vi "Begin.vi"(8 "error in":errorcluster) -> (0 "error out":errorcluster)   [LabVIEW 2020]
doc: "Called before other user functions, this VI is expected to open initial I/O refnums, load in file data, and do all program initialization. Notice that the <B>error out</B> terminal is simply used for data flow. Wiring it to other structures or subVIs ensures that this VI runs first."
uses:
  <vilib>/Rock Robotics/WPI/DriverStation/WPI_DriverStationRobotMode2.ctl
  <vilib>/Rock Robotics/WPI/Joystick/WPI_JoystickDeviceEnum.ctl
  <vilib>/Rock Robotics/WPI/ThirdParty/REV Robotics/REVLib/Typedef/Spark MAX Sensor Type.ctl
  Robot Global Data.vi
  <vilib>/Rock Robotics/Network Tables/NT Write String Array.vi
panel:
  in  "Steering BR PIDF":T1={"P Gain"=0.0, "I Gain"=0.0, "D Gain"=0.0, "F Gain"=0.0, "I Zone"=0.0, "Min Output"=-1.0, "Max Output"=1.0}
  in  "Steering BL PIDF":T1={"P Gain"=0.0, "I Gain"=0.0, "D Gain"=0.0, "F Gain"=0.0, "I Zone"=0.0, "Min Output"=-1.0, "Max Output"=1.0}
  in  "Steering FR PIDF":T1={"P Gain"=0.0, "I Gain"=0.0, "D Gain"=0.0, "F Gain"=0.0, "I Zone"=0.0, "Min Output"=-1.0, "Max Output"=1.0}
  in  "Steering FL PIDF":T1={"P Gain"=0.0, "I Gain"=0.0, "D Gain"=0.0, "F Gain"=0.0, "I Zone"=0.0, "Min Output"=-1.0, "Max Output"=1.0}
  in  "FR Zero":dbl
  in  "FL Zero":dbl
  in  "Reset Encoders":bool
  in  "BL Zero":dbl
  in  "BR Zero":dbl
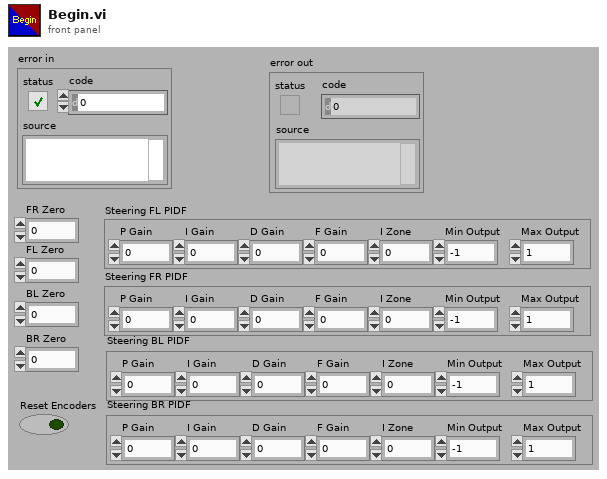
[diagram p1: front panel]
types:
  T1 = cluster{"P Gain":dbl, "I Gain":dbl, "D Gain":dbl, "F Gain":dbl, "I Zone":dbl, "Min Output":dbl, "Max Output":dbl}
  T2 = typedef "Spark MAX Sensor Type.ctl" = enum16{"No Sensor", "Hall Sensor", "Encoder", "-Not Available-", "Analog", "Alternate Encoder", "Duty Cycle"}
  T3 = typedef "WPI_JoystickDeviceEnum.ctl" = enum16{"USB 0", "USB 1", "USB 2", "USB 3", "USB 4", "USB 5"}
  T4 = typedef "WPI_DriverStationRobotMode2.ctl" = enum16{"Autonomous Disabled", "Autonomous Enabled", "Teleop Disabled", "Teleop Enabled", "Disconnected", "Finish", "Test Disabled", "Test Enabled", "Emergency Stopped"}
  T5 = typedef "WPI_JoystickDevRef.ctl" = cluster{"Device":T3}
  T6 = typedef "WPI_MotorControlDeviceRef.ctl" = cluster{"DeviceStatus":errorcluster, "Type":T7, "PWM":cluster{"PWM Channel":T8, "DeadBand":T9}, "CAN":cluster{"Device Number":u8, "SetOutput VI Ref":variant, "GetOutput VI Ref":variant, "Enable VI Ref":variant, "Disable VI Ref":variant, "Data":variant}, "Invert":bool, "DIO PWM":cluster{"PWM \"Enable\" Channel":T8, "DIOChannel":T10, "PWM Rate":dbl}}
  T7 = typedef "WPI_MotorControlType.ctl" = enum16{"PWM", "CAN", "DIO PWM"}
  T8 = typedef "FPGA_DIOPWMChannel.ctl" = enum8{"PWM 0", "PWM 1", "PWM 2", "PWM 3", "PWM 4", "PWM 5", "PWM 6", "PWM 7", "PWM 8", "PWM 9", "PWM MXP 0", "PWM MXP 1", "PWM MXP 2", "PWM MXP 3", "PWM MXP 4", "PWM MXP 5", "PWM MXP 6", "PWM MXP 7", "PWM MXP 8", "PWM MXP 9", "Invalid"}
  T9 = typedef "WPI_PWMDeadband.ctl" = cluster{"Name":string, "maxPositivePwm":i32, "minPositivePwm":i32, "centerPwm":i32, "maxNegativePwm":i32, "minNegativePwm":i32, "angularRange":u16}
  T10 = typedef "FPGA_DIOChannel.ctl" = enum8{"DIO 0", "DIO 1", "DIO 2", "DIO 3", "DIO 4", "DIO 5", "DIO 6", "DIO 7", "DIO 8", "DIO 9", "DIO MXP 0", "DIO MXP 1", "DIO MXP 2", "DIO MXP 3", "DIO MXP 4", "DIO MXP 5", "DIO MXP 6", "DIO MXP 7", "DIO MXP 8", "DIO MXP 9", "DIO MXP 10", "DIO MXP 11", "DIO MXP 12", "DIO MXP 13", "DIO MXP 14", "DIO MXP 15", "SPI Port CS1", "SPI Port CS2", "SPI Port CS3", "SPI Port MISO", "SPI Port MOSI", "Invalid"}
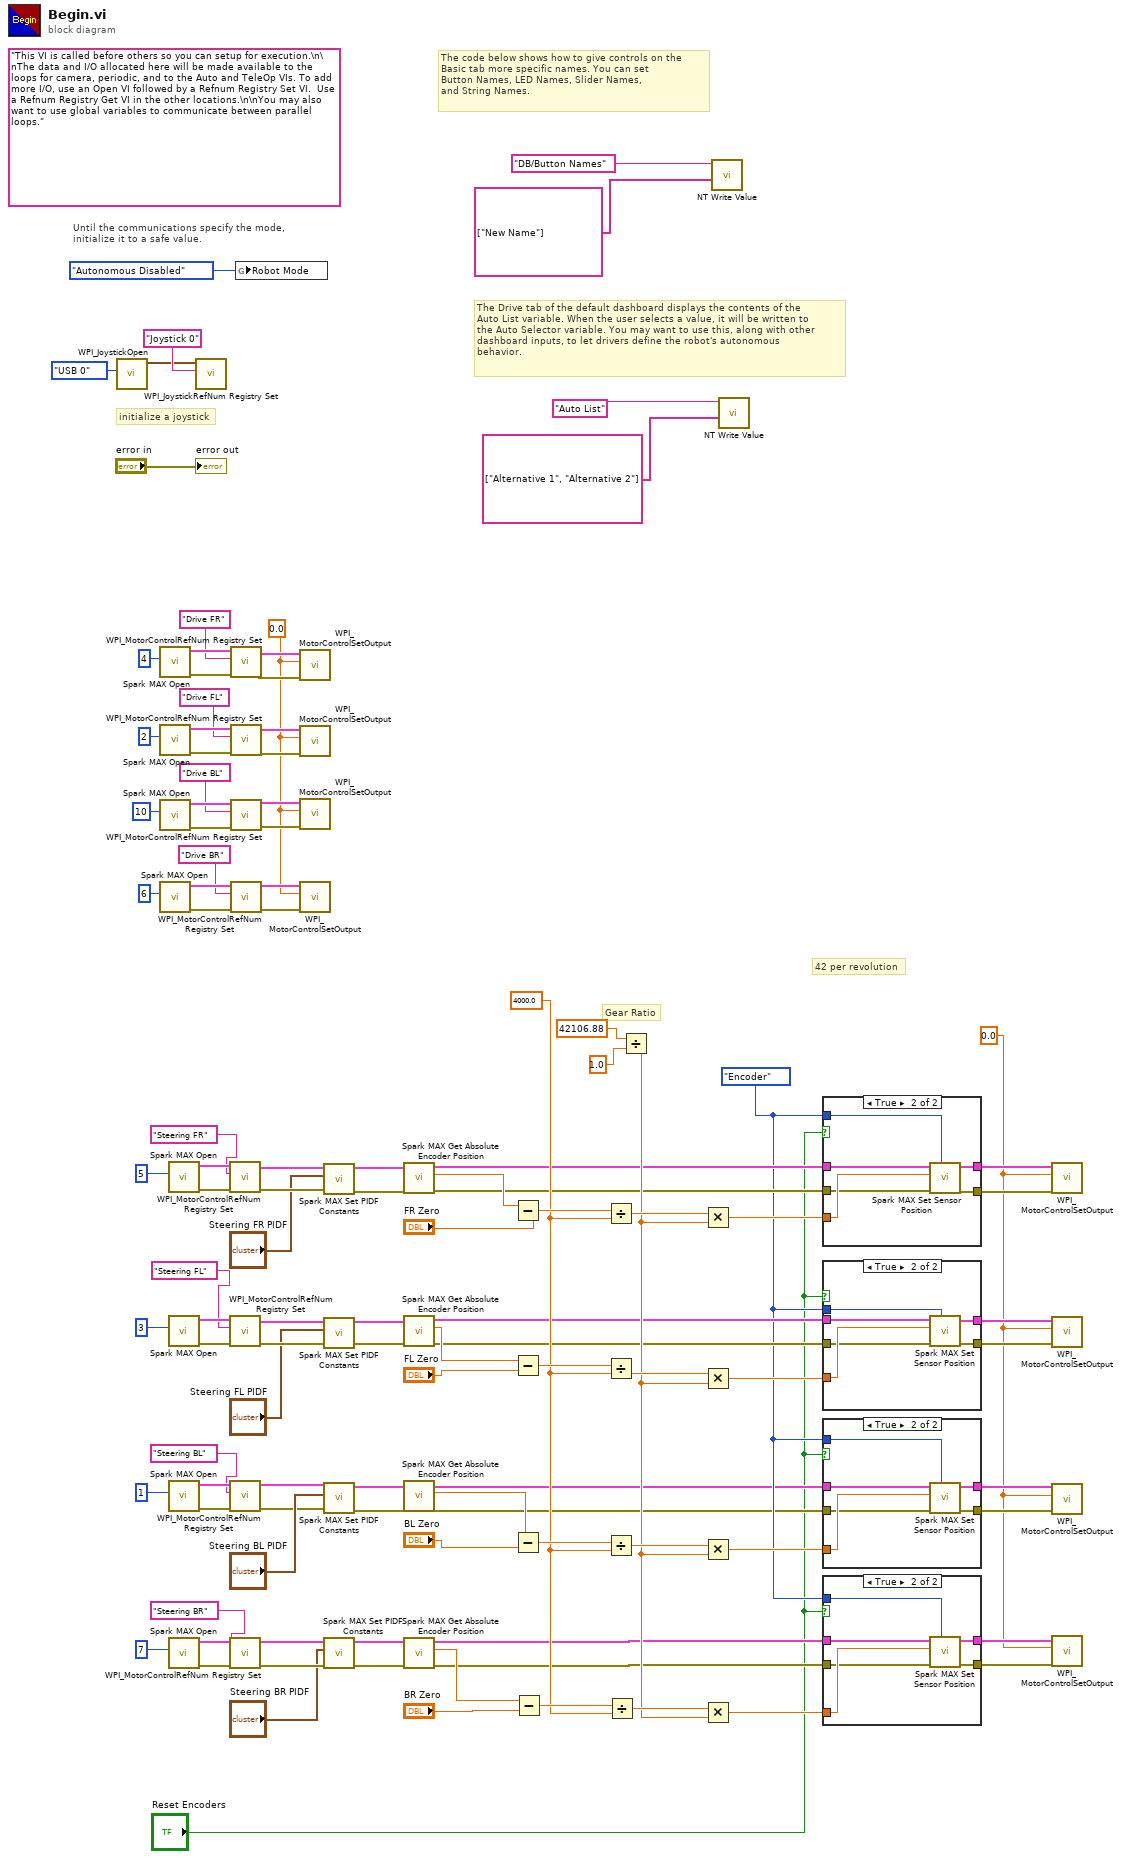
[diagram p0: block diagram]
diagram:
  w20 = 0.0 ("Output")
  w32 = Spark_MAX_Sensor_Type."Encoder" ("Sensor Type (Hall Sensor)")
  w43 = 4000.0 ("y")
  w79 = 0.0 ("Output")
  (unwired) "This VI is called before others so you can setup for execution.\n\nThe data and I/O allocated here will be made available to the loops for camera, periodic, and to the Auto and TeleOp VIs. To add more I/O, use an Open VI followed by a Refnum Registry Set VI.  Use a Refnum Registry Get VI in the other locations.\n\nYou may also want to use global variables to communicate between parallel loops."
  # "42 per revolution"
  # "Gear Ratio"
  # "The Drive tab of the default dashboard displays the contents of the\nAuto List variable. When the user selects a value, it will be written to\nthe Auto Selector variable. You may want to use this, along with other\ndashboard inputs, to let drivers define the robot's autonomous\nbehavior."
  # "The code below shows how to give controls on the\nBasic tab more specific names. You can set\nButton Names, LED Names, Slider Names,\nand String Names."
  # "initialize a joystick"
  # "Until the communications specify the mode,\ninitialize it to a safe value."
  n1 = call <vilib>:"WPI_JoystickOpen.vi"("JoystickDevice"=WPI_JoystickDeviceEnum."USB 0") -> ("JoystickDevRef"=w110:T5)  [unwired: 10 in]
  n2 = call <vilib>:"Spark MAX Open.vi"("Device Number"=u8 4) -> ("error out"=w102:errorcluster, "MotorControlDeviceRef"=w103:T6)  [unwired: 9 in]
  n3 = call <vilib>:"Spark MAX Open.vi"("Device Number"=u8 2) -> ("error out"=w98:errorcluster, "MotorControlDeviceRef"=w99:T6)  [unwired: 9 in]
  n4 = call <vilib>:"Spark MAX Open.vi"("Device Number"=u8 10) -> ("error out"=w94:errorcluster, "MotorControlDeviceRef"=w95:T6)  [unwired: 9 in]
  n5 = call <vilib>:"Spark MAX Open.vi"("Device Number"=u8 6) -> ("error out"=w90:errorcluster, "MotorControlDeviceRef"=w91:T6)  [unwired: 9 in]
  n6 = call <vilib>:"Spark MAX Open.vi"("Device Number"=u8 5) -> ("error out"=w77:errorcluster, "MotorControlDeviceRef"=w78:T6)  [unwired: 9 in]
  n7 = call <vilib>:"Spark MAX Open.vi"("Device Number"=u8 3) -> ("error out"=w73:errorcluster, "MotorControlDeviceRef"=w74:T6)  [unwired: 9 in]
  n8 = call <vilib>:"Spark MAX Open.vi"("Device Number"=u8 1) -> ("error out"=w69:errorcluster, "MotorControlDeviceRef"=w70:T6)  [unwired: 9 in]
  n9 = call <vilib>:"Spark MAX Open.vi"("Device Number"=u8 7) -> ("error out"=w65:errorcluster, "MotorControlDeviceRef"=w66:T6)  [unwired: 9 in]
  n10 = call <vilib>:"WPI_JoystickRefNum Registry Set.vi"("refnum name"="Joystick 0", "JoystickDevRef"=w110) -> ()  [unwired: 8 in, 2 out]
  n11 = call <vilib>:"WPI_MotorControlRefNum Registry Set.vi"("error in (no error)"=w77, "refnum name"="Steering FR", "MotorControlDevRef"=w78) -> ("error out"=w14:errorcluster, "MotorControlDevRef"=w15:T6)  [unwired: 7 in]
  n12 = call <vilib>:"WPI_MotorControlRefNum Registry Set.vi"("error in (no error)"=w73, "refnum name"="Steering FL", "MotorControlDevRef"=w74) -> ("error out"=w27:errorcluster, "MotorControlDevRef"=w17:T6)  [unwired: 7 in]
  n13 = call <vilib>:"WPI_MotorControlRefNum Registry Set.vi"("error in (no error)"=w69, "refnum name"="Steering BL", "MotorControlDevRef"=w70) -> ("error out"=w8:errorcluster, "MotorControlDevRef"=w9:T6)  [unwired: 7 in]
  n14 = call <vilib>:"WPI_MotorControlRefNum Registry Set.vi"("error in (no error)"=w65, "refnum name"="Steering BR", "MotorControlDevRef"=w66) -> ("error out"=w3:errorcluster, "MotorControlDevRef"=w2:T6)  [unwired: 7 in]
  n15 = call <vilib>:"WPI_MotorControlRefNum Registry Set.vi"("error in (no error)"=w102, "refnum name"="Drive FR", "MotorControlDevRef"=w103) -> ("error out"=w85:errorcluster, "MotorControlDevRef"=w84:T6)  [unwired: 7 in]
  n16 = call <vilib>:"WPI_MotorControlRefNum Registry Set.vi"("error in (no error)"=w98, "refnum name"="Drive FL", "MotorControlDevRef"=w99) -> ("error out"=w86:errorcluster, "MotorControlDevRef"=w87:T6)  [unwired: 7 in]
  n17 = call <vilib>:"WPI_MotorControlRefNum Registry Set.vi"("error in (no error)"=w94, "refnum name"="Drive BL", "MotorControlDevRef"=w95) -> ("error out"=w82:errorcluster, "MotorControlDevRef"=w83:T6)  [unwired: 7 in]
  n18 = call <vilib>:"WPI_MotorControlRefNum Registry Set.vi"("error in (no error)"=w90, "refnum name"="Drive BR", "MotorControlDevRef"=w91) -> ("error out"=w81:errorcluster, "MotorControlDevRef"=w80:T6)  [unwired: 7 in]
  n19 = global write "Robot Global Data.vi" "Robot Mode"(WPI_DriverStationRobotMode2."Autonomous Disabled" ("Robot Mode")) -> ()
  n20 = call <vilib>:"WPI_MotorControlSetOutput.vi"("error in (no error)"=w85, "Output"=w79, "MotorControlDevRef"=w84) -> ()  [unwired: 6 in, 3 out]
  n21 = call <vilib>:"WPI_MotorControlSetOutput.vi"("error in (no error)"=w86, "Output"=w79, "MotorControlDevRef"=w87) -> ()  [unwired: 6 in, 3 out]
  n22 = call <vilib>:"WPI_MotorControlSetOutput.vi"("error in (no error)"=w82, "Output"=w79, "MotorControlDevRef"=w83) -> ()  [unwired: 6 in, 3 out]
  n23 = call <vilib>:"WPI_MotorControlSetOutput.vi"("error in (no error)"=w81, "Output"=w79, "MotorControlDevRef"=w80) -> ()  [unwired: 6 in, 3 out]
  n24 = call <vilib>:"Spark MAX Set PIDF Constants.vi"("error in"=w14, "PID Constants"="Steering FR PIDF", "MotorControlDeviceRef"=w15) -> ("error out"=w13:errorcluster, "MotorControlDeviceRef"=w12:T6)  [unwired: 7 in]
  n25 = call <vilib>:"Spark MAX Set PIDF Constants.vi"("PID Constants"="Steering FL PIDF", "MotorControlDeviceRef"=w17) -> ("MotorControlDeviceRef"=w16:T6)  [unwired: 8 in, 1 out]
  n26 = call <vilib>:"Spark MAX Set PIDF Constants.vi"("error in"=w8, "PID Constants"="Steering BL PIDF", "MotorControlDeviceRef"=w9) -> ("error out"=w7:errorcluster, "MotorControlDeviceRef"=w6:T6)  [unwired: 7 in]
  n27 = call <vilib>:"Spark MAX Set PIDF Constants.vi"("error in"=w3, "PID Constants"="Steering BR PIDF", "MotorControlDeviceRef"=w2) -> ("error out"=w4:errorcluster, "MotorControlDeviceRef"=w5:T6)  [unwired: 7 in]
  n28 = call <vilib>:"Spark MAX Get Absolute Encoder Position.vi"("error in (no error)"=w13, "MotorControlDeviceRef in"=w12) -> ("error out"=w36:errorcluster, "Position"=w40:dbl, "MotorControlDeviceRef out"=w35:T6)  [unwired: 6 in, 1 out]
  n29 = call <vilib>:"Spark MAX Get Absolute Encoder Position.vi"("error in (no error)"=w27, "MotorControlDeviceRef in"=w16) -> ("error out"=w33:errorcluster, "Position"=w41:dbl, "MotorControlDeviceRef out"=w34:T6)  [unwired: 6 in, 1 out]
  n30 = call <vilib>:"Spark MAX Get Absolute Encoder Position.vi"("error in (no error)"=w7, "MotorControlDeviceRef in"=w6) -> ("error out"=w30:errorcluster, "Position"=w53:dbl, "MotorControlDeviceRef out"=w31:T6)  [unwired: 6 in, 1 out]
  n31 = call <vilib>:"Spark MAX Get Absolute Encoder Position.vi"("error in (no error)"=w4, "MotorControlDeviceRef in"=w5) -> ("error out"=w28:errorcluster, "Position"=w60:dbl, "MotorControlDeviceRef out"=w29:T6)  [unwired: 6 in, 1 out]
  n32 = Subtract(x=w40, y="FR Zero") -> (x-y=w48:dbl)
  n33 = Subtract(x=w41, y="FL Zero") -> (x-y=w50:dbl)
  n34 = Subtract(x=w53, y="BL Zero") -> (x-y=w55:dbl)
  n35 = Subtract(x=w60, y="BR Zero") -> (x-y=w62:dbl)
  n36 = Divide(x=w48, y=w43) -> (x/y=w47:dbl)
  n37 = Divide(x=w50, y=w43) -> (x/y=w49:dbl)
  n38 = Divide(x=w55, y=w43) -> (x/y=w54:dbl)
  n39 = Divide(x=w62, y=w43) -> (x/y=w61:dbl)
  n40 = Divide(x=42106.88 ("y"), y=1.0) -> (x/y=w44:dbl)
  n41 = Multiply(x=w47, y=w44) -> (x*y=w45:dbl)
  n42 = Multiply(x=w49, y=w44) -> (x*y=w46:dbl)
  n43 = Multiply(x=w54, y=w44) -> (x*y=w51:dbl)
  n44 = Multiply(x=w61, y=w44) -> (x*y=w59:dbl)
  n45 = call-poly <vilib>:"NT Write Value.vi"("value"=string[] ["New Name"], "name"="DB/Button Names" ("Name")) -> ()  [unwired: 9 in, 1 out]
  n46 = call-poly <vilib>:"NT Write Value.vi"("value"=string[] ["Alternative 1", "Alternative 2"] ("String Array"), "name"="Auto List" ("Name")) -> ()  [unwired: 9 in, 1 out]
  n47 = case shown="True" "Reset Encoders" {
    tunnel: w45 -> [_ w120]
    tunnel: [w114 w119] -> w38
    tunnel: [w113 w118] -> w37
    tunnel: w35 -> [w114 w117]
    tunnel: w36 -> [w113 w116]
    tunnel: w32 -> [_ w115]
    frame False {
    }
    frame True {
      n48 = call <vilib>:"Spark MAX Set Sensor Position.vi"("Sensor Type (Hall Sensor)"=w115, "error in"=w116, "Position"=w120, "MotorControlDeviceRef"=w117) -> ("error out"=w118:errorcluster, "MotorControlDeviceRef"=w119:T6)  [unwired: 6 in]
    }
  }
  n49 = case shown="True" "Reset Encoders" {
    tunnel: w46 -> [_ w128]
    tunnel: w34 -> [w122 w127]
    tunnel: w33 -> [w121 w126]
    tunnel: w32 -> [_ w125]
    tunnel: [w122 w124] -> w22
    tunnel: [w121 w123] -> w21
    frame False {
    }
    frame True {
      n50 = call <vilib>:"Spark MAX Set Sensor Position.vi"("Sensor Type (Hall Sensor)"=w125, "error in"=w126, "Position"=w128, "MotorControlDeviceRef"=w127) -> ("error out"=w123:errorcluster, "MotorControlDeviceRef"=w124:T6)  [unwired: 6 in]
    }
  }
  n51 = case shown="True" "Reset Encoders" {
    tunnel: w51 -> [_ w136]
    tunnel: w32 -> [_ w135]
    tunnel: w31 -> [w130 w134]
    tunnel: w30 -> [w129 w133]
    tunnel: [w130 w132] -> w24
    tunnel: [w129 w131] -> w23
    frame False {
    }
    frame True {
      n52 = call <vilib>:"Spark MAX Set Sensor Position.vi"("Sensor Type (Hall Sensor)"=w135, "error in"=w133, "Position"=w136, "MotorControlDeviceRef"=w134) -> ("error out"=w131:errorcluster, "MotorControlDeviceRef"=w132:T6)  [unwired: 6 in]
    }
  }
  n53 = case shown="True" "Reset Encoders" {
    tunnel: w59 -> [_ w144]
    tunnel: w32 -> [_ w143]
    tunnel: w29 -> [w138 w142]
    tunnel: w28 -> [w137 w141]
    tunnel: [w138 w140] -> w26
    tunnel: [w137 w139] -> w25
    frame False {
    }
    frame True {
      n54 = call <vilib>:"Spark MAX Set Sensor Position.vi"("Sensor Type (Hall Sensor)"=w143, "error in"=w141, "Position"=w144, "MotorControlDeviceRef"=w142) -> ("error out"=w139:errorcluster, "MotorControlDeviceRef"=w140:T6)  [unwired: 6 in]
    }
  }
  n55 = call <vilib>:"WPI_MotorControlSetOutput.vi"("error in (no error)"=w37, "Output"=w20, "MotorControlDevRef"=w38) -> ()  [unwired: 6 in, 3 out]
  n56 = call <vilib>:"WPI_MotorControlSetOutput.vi"("error in (no error)"=w21, "Output"=w20, "MotorControlDevRef"=w22) -> ()  [unwired: 6 in, 3 out]
  n57 = call <vilib>:"WPI_MotorControlSetOutput.vi"("error in (no error)"=w23, "Output"=w20, "MotorControlDevRef"=w24) -> ()  [unwired: 6 in, 3 out]
  n58 = call <vilib>:"WPI_MotorControlSetOutput.vi"("error in (no error)"=w25, "Output"=w20, "MotorControlDevRef"=w26) -> ()  [unwired: 6 in, 3 out]
  "error out" <- "error in"
